vi "Hall_analysis_dataview.vi"(8 "Y-column names":string[](array[string])=["Kxy"], 10 "column extension":string[](array[string])=["NC", "C"], 11 "Graph array":cluster{"output":dbl[], "output":dbl[]}[](array[cluster])=[{"output"=[-18.0, -17.8, -17.5, -17.2, -16.9, -16.6, -16.3, -16.0, -15.7, -15.4, -15.1, -14.8, -14.5, -14.2, -13.9, -13.6, -13.3, -13.0, -12.7, -12.4, -12.1, -11.8, -11.5, -11.2, -10.9, -10.6, -10.3, -10.0, -9.7, -9.4, -9.2, -9.0, -8.8, -8.6, -8.4, -8.2, -8.0, -7.8, -7.6, -7.4, -7.2, -7.0, -6.8, -6.6, -6.4, -6.2, -6.0, -5.8, -5.6, -5.4, -5.2, -5.0, -4.8, -4.6, -4.4, -4.2, -4.1, -4.0, -3.9, -3.8, -3.7, -3.6, -3.5, -3.4, -3.3, -3.2, -3.1, -3.0, -2.9, -2.8, -2.7, -2.6, -2.5, -2.4, -2.3, -2.2, -2.1, -2.0, -1.9, -1.8, -1.7, -1.6, -1.5, -1.4, -1.3, -1.2, -1.1, -1.0, -0.9, -0.8, -0.7, -0.6, -0.5, -0.4, -0.3, -0.2, -0.1, 0.0, 0.1, 0.2, 0.3, 0.4, 0.5, 0.6, 0.6, 0.7, 0.7, 0.8, 0.8, 0.9, 0.9, 1.0, 1.0, 1.1, 1.1, 1.2, 1.2, 1.3, 1.3, 1.4, 1.4, 1.5, 1.5, 1.6, 1.6, 1.7, 1.7, 1.8, 1.8, 1.9, 1.9, 1.9, 2.0, 2.0, 2.0, 2.0, 2.1, 2.2, 2.3, 2.4, 2.5, 2.6, 2.7, 2.8, 2.9, 3.0, 3.1, 3.2, 3.3, 3.4, 3.5, 3.6, 3.7, 3.8, 3.9, 4.0, 4.1, 4.3, 4.5, 4.7, 4.9, 5.1, 5.3, 5.5, 5.7, 5.9, 6.1, 6.3, 6.5, 6.7, 6.9, 7.1, 7.3, 7.5, 7.7, 7.9, 8.1, 8.3, 8.5, 8.7, 8.9, 9.1, 9.3, 9.6, 9.9, 10.2, 10.5, 11.4, 11.7, 12.0, 12.3, 12.6, 12.9, 13.2, 13.5, 13.8, 14.1, 14.4, 14.7, 15.0, 15.3, 15.6, 15.9, 16.2, 16.5, 16.8, 17.1, 17.4, 17.7, 18.0], "output"=[0.054529, 0.058942, 0.066239, 0.077061, 0.087056, 0.10131, 0.11992, 0.1396, 0.16271, 0.18625, 0.2129, 0.23568, 0.26388, 0.29975, 0.34124, 0.37943, 0.3989, 0.44212, 0.48919, 0.5041, 0.54167, 0.58119, 0.59731, 0.60919, 0.66613, 0.66507, 0.71084, 0.72607, 0.72221, 0.74336, 0.77984, 0.77621, 0.77261, 0.80307, 0.76644, 0.80808, 0.81198, 0.81508, 0.79026, 0.84278, 0.81013, 0.81826, 0.84746, 0.83187, 0.83075, 0.83154, 0.81118, 0.84682, 0.85035, 0.83341, 0.83691, 0.79145, 0.83157, 0.83834, 0.80534, 0.81804, 0.82836, 0.82435, 0.78641, 0.75032, 0.7595, 0.77179, 0.77151, 0.778, 0.80644, 0.74695, 0.74781, 0.74014, 0.79086, 0.72817, 0.75592, 0.74425, 0.74898, 0.73582, 0.73516, 0.72155, 0.71542, 0.71347, 0.73071, 0.70282, 0.69885, 0.70647, 0.70025, 0.67747, 0.68127, 0.70861, 0.67626, 0.68964, 0.64825, 0.67411, 0.66336, 0.656, 0.65756, 0.67107, 0.70006, 0.698, 0.67342, 0.6801, 0.66464, 0.63203, 0.69444, 0.708, 0.69388, 0.7146, 0.66843, 0.74125, 0.64612, 0.73964, 0.62851, 0.7537, 0.66641, 0.72491, 0.69419, 0.73232, 0.67301, 0.72483, 0.68845, 0.76522, 0.69356, 0.72033, 0.67263, 0.73855, 0.67125, 0.77098, 0.74016, 0.74964, 0.69619, 0.77965, 0.75816, 0.76918, 0.73759, 0.77935, 0.78748, 0.81876, 0.77574, 0.73471, 0.81422, 0.78848, 0.82829, 0.80536, 0.78947, 0.79377, 0.78297, 0.81896, 0.83866, 0.84293, 0.84248, 0.85276, 0.85255, 0.83921, 0.86151, 0.84402, 0.87765, 0.84703, 0.84606, 0.86928, 0.83403, 0.86374, 0.84952, 0.87353, 0.85058, 0.86321, 0.84461, 0.88025, 0.872, 0.89059, 0.88649, 0.888, 0.88664, 0.86834, 0.88418, 0.87369, 0.82698, 0.83785, 0.8636, 0.86849, 0.84876, 0.84895, 0.86216, 0.85159, 0.77613, 0.81179, 0.80194, 0.77828, 0.80233, 0.73352, 0.7213, 0.63859, 0.62626, 0.60173, 0.57119, 0.51729, 0.48595, 0.42536, 0.4044, 0.36236, 0.32568, 0.28429, 0.25023, 0.22166, 0.19862, 0.1831, 0.14912, 0.12865, 0.11025, 0.094853, 0.081756, 0.070731, 0.062495, 0.055254]}, {"output"=[-18.0, -17.8, -17.5, -17.2, -16.9, -16.6, -16.3, -16.0, -15.7, -15.4, -15.1, -14.8, -14.5, -14.2, -13.9, -13.6, -13.3, -13.0, -12.7, -12.4, -12.1, -11.8, -11.5, -11.2, -10.9, -10.6, -10.3, -10.0, -9.7, -9.4, -9.2, -9.0, -8.8, -8.6, -8.4, -8.2, -8.0, -7.8, -7.6, -7.4, -7.2, -7.0, -6.8, -6.6, -6.4, -6.2, -6.0, -5.8, -5.6, -5.4, -5.2, -5.0, -4.8, -4.6, -4.4, -4.2, -4.1, -4.0, -3.9, -3.8, -3.7, -3.6, -3.5, -3.4, -3.3, -3.2, -3.1, -3.0, -2.9, -2.8, -2.7, -2.6, -2.5, -2.4, -2.3, -2.2, -2.1, -2.0, -1.9, -1.8, -1.7, -1.6, -1.5, -1.4, -1.3, -1.2, -1.1, -1.0, -0.9, -0.8, -0.7, -0.6, -0.5, -0.4, -0.3, -0.2, -0.1, 0.0, 0.0, 0.0, 0.0, 0.1, 0.1, 0.2, 0.2, 0.3, 0.3, 0.4, 0.4, 0.5, 0.5, 0.6, 0.6, 0.7, 0.7, 0.8, 0.8, 0.9, 0.9, 1.0, 1.0, 1.1, 1.1, 1.2, 1.2, 1.2, 1.3, 1.4, 1.4, 1.4, 1.5, 1.5, 1.5, 1.6, 1.6, 1.6, 1.7, 1.7, 1.7, 1.8, 1.8, 1.8, 1.9, 1.9, 1.9, 1.9, 2.0, 2.0, 2.0, 2.0, 2.0, 2.1, 2.2, 2.3, 2.4, 2.5, 2.6, 2.7, 2.8, 2.9, 3.0, 3.2, 3.3, 3.4, 3.5, 3.6, 3.7, 3.8, 3.9, 4.0, 4.1, 4.3, 4.5, 4.7, 4.9, 5.1, 5.3, 5.5, 5.7, 5.9, 6.1, 6.3, 6.5, 6.7, 6.9, 7.1, 7.3, 7.5, 7.7, 7.9, 8.1, 8.3, 8.5, 8.7, 8.9, 9.1, 9.3, 9.6, 9.9, 10.2, 10.5, 11.4, 11.7, 12.0, 12.3, 12.6, 12.9, 13.2, 13.5, 13.8, 14.1, 14.4, 14.7, 15.0, 15.3, 15.6, 15.9, 16.2, 16.5, 16.8, 17.1, 17.4, 17.7, 18.0], "output"=[0.04639503, 0.05124551, 0.05869006, 0.06889321, 0.07842688, 0.09168241, 0.1088334, 0.1275547, 0.1497657, 0.1728078, 0.1996734, 0.2230474, 0.252526, 0.2881616, 0.327736, 0.3626875, 0.3799339, 0.4162642, 0.4502874, 0.4540727, 0.4752561, 0.4913592, 0.4877077, 0.4808698, 0.5060909, 0.4841805, 0.4946125, 0.4869426, 0.4643427, 0.4633326, 0.475855, 0.4651067, 0.45418, 0.4655186, 0.439674, 0.4540213, 0.4526447, 0.452366, 0.4296351, 0.4631344, 0.4392119, 0.4478341, 0.4652855, 0.4548735, 0.4575837, 0.4587661, 0.4438654, 0.469387, 0.470055, 0.4578611, 0.4516406, 0.4175235, 0.436408, 0.4269168, 0.3872179, 0.3819697, 0.3767659, 0.3588841, 0.3260986, 0.2882154, 0.2814761, 0.2736725, 0.2563214, 0.2451817, 0.2437467, 0.1887873, 0.1645303, 0.1499105, 0.1638911, 0.1060275, 0.09419492, 0.06499817, 0.0570674, 0.02551558, 0.003708405, -0.02605604, -0.04799681, -0.06751369, -0.0846491, -0.1206419, -0.146525, -0.1597774, -0.1865335, -0.2201835, -0.2416687, -0.2474123, -0.2807871, -0.295045, -0.3360811, -0.3413561, -0.3589792, -0.3818877, -0.3994011, -0.4013593, -0.398709, -0.4129966, -0.4294426, -0.4040814, -0.4025437, -0.3969354, -0.4430137, -0.3701796, -0.4330835, -0.3728167, -0.4410564, -0.3769775, -0.400408, -0.3534563, -0.3830965, -0.3413242, -0.3789024, -0.3517245, -0.3759194, -0.3247219, -0.3729292, -0.3118913, -0.3624734, -0.2877669, -0.3256675, -0.2765885, -0.2927328, -0.2603341, -0.2851914, -0.2416307, -0.2405671, -0.2581909, -0.2354419, -0.1993335, -0.1469915, -0.2259791, -0.1720161, -0.3363505, -0.2092051, -0.1346528, -0.03116894, -0.1574943, -0.1216288, -0.2430438, -0.1582942, -0.08931337, -0.1297527, -0.1192861, -0.07149084, -0.1419238, -0.1457252, -0.09284115, -0.03720788, -0.102183, -0.1086995, -0.04796695, -0.104636, -0.00174423, 0.009173533, 0.05047776, 0.05254663, 0.07652015, 0.08893176, 0.1113383, 0.151861, 0.1836534, 0.1970177, 0.2455877, 0.2636115, 0.2712736, 0.3057058, 0.3097401, 0.3473493, 0.3425707, 0.3539546, 0.3803674, 0.3816536, 0.4126079, 0.4150657, 0.4464129, 0.44045, 0.4582221, 0.4505175, 0.4758656, 0.4795104, 0.4947396, 0.4848849, 0.4830822, 0.4786933, 0.4679154, 0.4795023, 0.4728305, 0.4473741, 0.4516747, 0.4679614, 0.4744294, 0.46412, 0.4744021, 0.487967, 0.4956767, 0.4472478, 0.4861927, 0.4899166, 0.4858326, 0.5285123, 0.5022734, 0.5113373, 0.5215333, 0.5057456, 0.4986291, 0.4954527, 0.4628171, 0.4464335, 0.3980344, 0.3780465, 0.3425009, 0.3082822, 0.2687738, 0.2353835, 0.2080937, 0.1842725, 0.1676573, 0.1364157, 0.1169751, 0.09968616, 0.0853419, 0.07318228, 0.06282505, 0.05469888, 0.0469797]}]) -> ()   [LabVIEW 2024]
uses:
  <vilib>/gmath/NI_Gmath.lvlib
panel:
  out "y-column name":string="Kxy_NCC"
  out "Hall data":cluster{"output":dbl[], "output":dbl[]}[](graph)=[{"output"=[-0.0, 0.3272743225097656, 0.6545467376708984, 0.9818191528320312, 1.309091567993164, 1.6363639831542969, 1.9636363983154297, 2.290909767150879, 2.6181821823120117, 2.945455551147461, 3.2727279663085938, 3.6000003814697266, 3.927273750305176, 4.254546165466309, 4.581818580627441, 4.909091949462891, 5.236364364624023, 5.563636779785156, 5.890909194946289, 6.218182563781738, 6.545454978942871, 6.872727394104004, 7.200000762939453, 7.527273178100586, 7.854545593261719, 8.181818962097168, 8.5090913772583, 8.836363792419434, 9.163637161254883, 9.490909576416016, 9.818181991577148, 10.145454406738281, 10.47272777557373, 10.800000190734863, 11.127273559570312, 11.454545974731445, 11.781818389892578, 12.109090805053711, 12.436363220214844, 12.763636589050293, 13.090909957885742, 13.418182373046875, 13.745454788208008, 14.07272720336914, 14.399999618530273, 14.727272987365723, 15.054545402526855, 15.381818771362305, 15.709091186523438, 16.03636360168457, 16.363636016845703, 16.690908432006836, 17.0181827545166, 17.345455169677734, 17.672727584838867, 18.0], "output"=[0.0, 0.00299248279571529, -0.0018767957687377823, 0.003511941719055167, 0.0053665068054198906, 0.010236265392303434, 0.008009093399047817, 0.04537398966789241, 0.022717283315658587, 0.03639796306610105, 0.031195704059600815, 0.03611515687942507, 0.027817319812774688, 0.021205686359405507, 0.012001070156097415, 0.020733940610885626, 0.007127333927154533, 0.01517751313209531, 0.029562425460815445, 0.027957046141624475, 0.025458204402923568, 0.02258906681060785, 0.020102571363449062, 0.016001556339263923, 0.026572024908065817, 0.020201597528457627, 0.037629742684364365, 0.01343787633895871, 0.014737974634170536, 0.024966436818440796, 0.03602008089701325, 0.013672806886037503, 0.018961714207331226, 0.013976701386769541, 0.020330128383636348, 0.018619129714965765, 0.018701590213775487, 0.025046611016591225, 0.022198663406372054, 0.010495055723190427, 0.009185015996297174, 0.009443247070312494, 0.004545132083892844, 0.005831363080342794, 0.0042268017514546785, 0.002558227068583274, 0.0005598068555196234, 0.003261120878855439, 0.004366964670816931, 0.0013005196634929411, 0.0013206059392292177, 0.001730701716105211, 0.0011047034600575323, 0.00046085776265467754, 0.0006030408445993653, 0.00036249999999999824]}, {"output"=[-0.0, 0.3272743225097656, 0.6545467376708984, 0.9818191528320312, 1.309091567993164, 1.6363639831542969, 1.9636363983154297, 2.290909767150879, 2.6181821823120117, 2.945455551147461, 3.2727279663085938, 3.6000003814697266, 3.927273750305176, 4.254546165466309, 4.581818580627441, 4.909091949462891, 5.236364364624023, 5.563636779785156, 5.890909194946289, 6.218182563781738, 6.545454978942871, 6.872727394104004, 7.200000762939453, 7.527273178100586, 7.854545593261719, 8.181818962097168, 8.5090913772583, 8.836363792419434, 9.163637161254883, 9.490909576416016, 9.818181991577148, 10.145454406738281, 10.47272777557373, 10.800000190734863, 11.127273559570312, 11.454545974731445, 11.781818389892578, 12.109090805053711, 12.436363220214844, 12.763636589050293, 13.090909957885742, 13.418182373046875, 13.745454788208008, 14.07272720336914, 14.399999618530273, 14.727272987365723, 15.054545402526855, 15.381818771362305, 15.709091186523438, 16.03636360168457, 16.363636016845703, 16.690908432006836, 17.0181827545166, 17.345455169677734, 17.672727584838867, 18.0], "output"=[0.0, 0.0018725577600479104, -0.0024482699415207254, 0.0018922374864578095, 0.0025667974205016986, -0.0168217872724533, -0.024209317914752962, 0.022859984019057276, 0.011349383976507185, 0.01609591005096435, 0.01496877274971009, 0.018033754336547858, 0.013058585019016272, 0.011085874159431464, 0.0022907896628856783, 0.007575240142726897, 9.869320383074087e-05, 0.004593664635086064, 0.018130483435058575, 0.012580532687187201, 0.010315582862472528, 0.009491347095203384, 0.010445227202796947, 0.00603945345125198, 0.010258666759109497, 0.007215023374080642, 0.01727315357503889, 0.0032452536701679524, 0.006738375054264056, 0.011839508860651687, 0.021813215582338813, 0.00819147609920512, 0.010953557992998797, 0.007974255379909978, 0.015729827381049277, 0.015995607844606963, 0.006333438585472084, 0.011429940308507275, 0.013502250313059488, 0.005405149334716863, 0.005189663690376267, 0.0051790019136429, 0.0016113218469619717, 0.0032211251384736683, 0.00218476138941448, 0.0013544852338791824, 0.00027394241498311656, 0.002652594708252007, 0.0036020352183022963, 0.0011468679021836292, 0.0011747290191267898, 0.0014462527038765494, 0.0009137086473528164, 0.0003810429619217487, 0.0005169348717689037, 0.0002923350000000012]}]
  in  "Data analyis method":T1(ring)
  in  "smooth":bool=TRUE
  in  "smooth factor":i32=1
  in  "iteration Number":i32=1
  in  "interpolation size":u16=111 min=1 step=1
  in  "max H":sgl=18.0 min=0 format="%.2f"
  in  "export":T2(ring)=enum."write to clipboard"
  out "raw data":cluster{"all rows":dbl[], "all rows":dbl[]}[](graph)=[{"all rows"=[-18.0, -17.8, -17.5, -17.2, -16.9, -16.6, -16.3, -16.0, -15.7, -15.4, -15.1, -14.8, -14.5, -14.2, -13.9, -13.6, -13.3, -13.0, -12.7, -12.4, -12.1, -11.8, -11.5, -11.2, -10.9, -10.6, -10.3, -10.0, -9.7, -9.4, -9.2, -9.0, -8.8, -8.6, -8.4, -8.2, -8.0, -7.8, -7.6, -7.4, -7.2, -7.0, -6.8, -6.6, -6.4, -6.2, -6.0, -5.8, -5.6, -5.4, -5.2, -5.0, -4.8, -4.6, -4.4, -4.2, -4.1, -4.0, -3.9, -3.8, -3.7, -3.6, -3.5, -3.4, -3.3, -3.2, -3.1, -3.0, -2.9, -2.8, -2.7, -2.6, -2.5, -2.4, -2.3, -2.2, -2.1, -2.0, -1.9, -1.8, -1.7, -1.6, -1.5, -1.4, -1.3, -1.2, -1.1, -1.0, -0.9, -0.8, -0.7, -0.6, -0.5, -0.4, -0.3, -0.2, -0.1, 0.0, 0.1, 0.2, 0.3, 0.4, 0.5, 0.6, 0.6, 0.7, 0.7, 0.8, 0.8, 0.9, 0.9, 1.0, 1.0, 1.1, 1.1, 1.2, 1.2, 1.3, 1.3, 1.4, 1.4, 1.5, 1.5, 1.6, 1.6, 1.7, 1.7, 1.8, 1.8, 1.9, 1.9, 1.9, 2.0, 2.0, 2.0, 2.0, 2.1, 2.2, 2.3, 2.4, 2.5, 2.6, 2.7, 2.8, 2.9, 3.0, 3.1, 3.2, 3.3, 3.4, 3.5, 3.6, 3.7, 3.8, 3.9, 4.0, 4.1, 4.3, 4.5, 4.7, 4.9, 5.1, 5.3, 5.5, 5.7, 5.9, 6.1, 6.3, 6.5, 6.7, 6.9, 7.1, 7.3, 7.5, 7.7, 7.9, 8.1, 8.3, 8.5, 8.7, 8.9, 9.1, 9.3, 9.6, 9.9, 10.2, 10.5, 11.4, 11.7, 12.0, 12.3, 12.6, 12.9, 13.2, 13.5, 13.8, 14.1, 14.4, 14.7, 15.0, 15.3, 15.6, 15.9, 16.2, 16.5, 16.8, 17.1, 17.4, 17.7, 18.0], "all rows"=[0.054529, 0.058942, 0.066239, 0.077061, 0.087056, 0.10131, 0.11992, 0.1396, 0.16271, 0.18625, 0.2129, 0.23568, 0.26388, 0.29975, 0.34124, 0.37943, 0.3989, 0.44212, 0.48919, 0.5041, 0.54167, 0.58119, 0.59731, 0.60919, 0.66613, 0.66507, 0.71084, 0.72607, 0.72221, 0.74336, 0.77984, 0.77621, 0.77261, 0.80307, 0.76644, 0.80808, 0.81198, 0.81508, 0.79026, 0.84278, 0.81013, 0.81826, 0.84746, 0.83187, 0.83075, 0.83154, 0.81118, 0.84682, 0.85035, 0.83341, 0.83691, 0.79145, 0.83157, 0.83834, 0.80534, 0.81804, 0.82836, 0.82435, 0.78641, 0.75032, 0.7595, 0.77179, 0.77151, 0.778, 0.80644, 0.74695, 0.74781, 0.74014, 0.79086, 0.72817, 0.75592, 0.74425, 0.74898, 0.73582, 0.73516, 0.72155, 0.71542, 0.71347, 0.73071, 0.70282, 0.69885, 0.70647, 0.70025, 0.67747, 0.68127, 0.70861, 0.67626, 0.68964, 0.64825, 0.67411, 0.66336, 0.656, 0.65756, 0.67107, 0.70006, 0.698, 0.67342, 0.6801, 0.66464, 0.63203, 0.69444, 0.708, 0.69388, 0.7146, 0.66843, 0.74125, 0.64612, 0.73964, 0.62851, 0.7537, 0.66641, 0.72491, 0.69419, 0.73232, 0.67301, 0.72483, 0.68845, 0.76522, 0.69356, 0.72033, 0.67263, 0.73855, 0.67125, 0.77098, 0.74016, 0.74964, 0.69619, 0.77965, 0.75816, 0.76918, 0.73759, 0.77935, 0.78748, 0.81876, 0.77574, 0.73471, 0.81422, 0.78848, 0.82829, 0.80536, 0.78947, 0.79377, 0.78297, 0.81896, 0.83866, 0.84293, 0.84248, 0.85276, 0.85255, 0.83921, 0.86151, 0.84402, 0.87765, 0.84703, 0.84606, 0.86928, 0.83403, 0.86374, 0.84952, 0.87353, 0.85058, 0.86321, 0.84461, 0.88025, 0.872, 0.89059, 0.88649, 0.888, 0.88664, 0.86834, 0.88418, 0.87369, 0.82698, 0.83785, 0.8636, 0.86849, 0.84876, 0.84895, 0.86216, 0.85159, 0.77613, 0.81179, 0.80194, 0.77828, 0.80233, 0.73352, 0.7213, 0.63859, 0.62626, 0.60173, 0.57119, 0.51729, 0.48595, 0.42536, 0.4044, 0.36236, 0.32568, 0.28429, 0.25023, 0.22166, 0.19862, 0.1831, 0.14912, 0.12865, 0.11025, 0.094853, 0.081756, 0.070731, 0.062495, 0.055254]}, {"all rows"=[-18.0, -17.8, -17.5, -17.2, -16.9, -16.6, -16.3, -16.0, -15.7, -15.4, -15.1, -14.8, -14.5, -14.2, -13.9, -13.6, -13.3, -13.0, -12.7, -12.4, -12.1, -11.8, -11.5, -11.2, -10.9, -10.6, -10.3, -10.0, -9.7, -9.4, -9.2, -9.0, -8.8, -8.6, -8.4, -8.2, -8.0, -7.8, -7.6, -7.4, -7.2, -7.0, -6.8, -6.6, -6.4, -6.2, -6.0, -5.8, -5.6, -5.4, -5.2, -5.0, -4.8, -4.6, -4.4, -4.2, -4.1, -4.0, -3.9, -3.8, -3.7, -3.6, -3.5, -3.4, -3.3, -3.2, -3.1, -3.0, -2.9, -2.8, -2.7, -2.6, -2.5, -2.4, -2.3, -2.2, -2.1, -2.0, -1.9, -1.8, -1.7, -1.6, -1.5, -1.4, -1.3, -1.2, -1.1, -1.0, -0.9, -0.8, -0.7, -0.6, -0.5, -0.4, -0.3, -0.2, -0.1, 0.0, 0.0, 0.0, 0.0, 0.1, 0.1, 0.2, 0.2, 0.3, 0.3, 0.4, 0.4, 0.5, 0.5, 0.6, 0.6, 0.7, 0.7, 0.8, 0.8, 0.9, 0.9, 1.0, 1.0, 1.1, 1.1, 1.2, 1.2, 1.2, 1.3, 1.4, 1.4, 1.4, 1.5, 1.5, 1.5, 1.6, 1.6, 1.6, 1.7, 1.7, 1.7, 1.8, 1.8, 1.8, 1.9, 1.9, 1.9, 1.9, 2.0, 2.0, 2.0, 2.0, 2.0, 2.1, 2.2, 2.3, 2.4, 2.5, 2.6, 2.7, 2.8, 2.9, 3.0, 3.2, 3.3, 3.4, 3.5, 3.6, 3.7, 3.8, 3.9, 4.0, 4.1, 4.3, 4.5, 4.7, 4.9, 5.1, 5.3, 5.5, 5.7, 5.9, 6.1, 6.3, 6.5, 6.7, 6.9, 7.1, 7.3, 7.5, 7.7, 7.9, 8.1, 8.3, 8.5, 8.7, 8.9, 9.1, 9.3, 9.6, 9.9, 10.2, 10.5, 11.4, 11.7, 12.0, 12.3, 12.6, 12.9, 13.2, 13.5, 13.8, 14.1, 14.4, 14.7, 15.0, 15.3, 15.6, 15.9, 16.2, 16.5, 16.8, 17.1, 17.4, 17.7, 18.0], "all rows"=[0.04639503, 0.05124551, 0.05869006, 0.06889321, 0.07842688, 0.09168241, 0.1088334, 0.1275547, 0.1497657, 0.1728078, 0.1996734, 0.2230474, 0.252526, 0.2881616, 0.327736, 0.3626875, 0.3799339, 0.4162642, 0.4502874, 0.4540727, 0.4752561, 0.4913592, 0.4877077, 0.4808698, 0.5060909, 0.4841805, 0.4946125, 0.4869426, 0.4643427, 0.4633326, 0.475855, 0.4651067, 0.45418, 0.4655186, 0.439674, 0.4540213, 0.4526447, 0.452366, 0.4296351, 0.4631344, 0.4392119, 0.4478341, 0.4652855, 0.4548735, 0.4575837, 0.4587661, 0.4438654, 0.469387, 0.470055, 0.4578611, 0.4516406, 0.4175235, 0.436408, 0.4269168, 0.3872179, 0.3819697, 0.3767659, 0.3588841, 0.3260986, 0.2882154, 0.2814761, 0.2736725, 0.2563214, 0.2451817, 0.2437467, 0.1887873, 0.1645303, 0.1499105, 0.1638911, 0.1060275, 0.09419492, 0.06499817, 0.0570674, 0.02551558, 0.003708405, -0.02605604, -0.04799681, -0.06751369, -0.0846491, -0.1206419, -0.146525, -0.1597774, -0.1865335, -0.2201835, -0.2416687, -0.2474123, -0.2807871, -0.295045, -0.3360811, -0.3413561, -0.3589792, -0.3818877, -0.3994011, -0.4013593, -0.398709, -0.4129966, -0.4294426, -0.4040814, -0.4025437, -0.3969354, -0.4430137, -0.3701796, -0.4330835, -0.3728167, -0.4410564, -0.3769775, -0.400408, -0.3534563, -0.3830965, -0.3413242, -0.3789024, -0.3517245, -0.3759194, -0.3247219, -0.3729292, -0.3118913, -0.3624734, -0.2877669, -0.3256675, -0.2765885, -0.2927328, -0.2603341, -0.2851914, -0.2416307, -0.2405671, -0.2581909, -0.2354419, -0.1993335, -0.1469915, -0.2259791, -0.1720161, -0.3363505, -0.2092051, -0.1346528, -0.03116894, -0.1574943, -0.1216288, -0.2430438, -0.1582942, -0.08931337, -0.1297527, -0.1192861, -0.07149084, -0.1419238, -0.1457252, -0.09284115, -0.03720788, -0.102183, -0.1086995, -0.04796695, -0.104636, -0.00174423, 0.009173533, 0.05047776, 0.05254663, 0.07652015, 0.08893176, 0.1113383, 0.151861, 0.1836534, 0.1970177, 0.2455877, 0.2636115, 0.2712736, 0.3057058, 0.3097401, 0.3473493, 0.3425707, 0.3539546, 0.3803674, 0.3816536, 0.4126079, 0.4150657, 0.4464129, 0.44045, 0.4582221, 0.4505175, 0.4758656, 0.4795104, 0.4947396, 0.4848849, 0.4830822, 0.4786933, 0.4679154, 0.4795023, 0.4728305, 0.4473741, 0.4516747, 0.4679614, 0.4744294, 0.46412, 0.4744021, 0.487967, 0.4956767, 0.4472478, 0.4861927, 0.4899166, 0.4858326, 0.5285123, 0.5022734, 0.5113373, 0.5215333, 0.5057456, 0.4986291, 0.4954527, 0.4628171, 0.4464335, 0.3980344, 0.3780465, 0.3425009, 0.3082822, 0.2687738, 0.2353835, 0.2080937, 0.1842725, 0.1676573, 0.1364157, 0.1169751, 0.09968616, 0.0853419, 0.07318228, 0.06282505, 0.05469888, 0.0469797]}]
  in  "stop":bool
  in  "export Hall data":bool
  # "Fitting is done for the range given by 'Bbkg init' and 'Bbkg final'.\nBackground curve is extended to the range give by 'B init' and 'B final'.\nFFT is done in the range given by 'B init' and 'B final'."
  # "Also removes NaN"
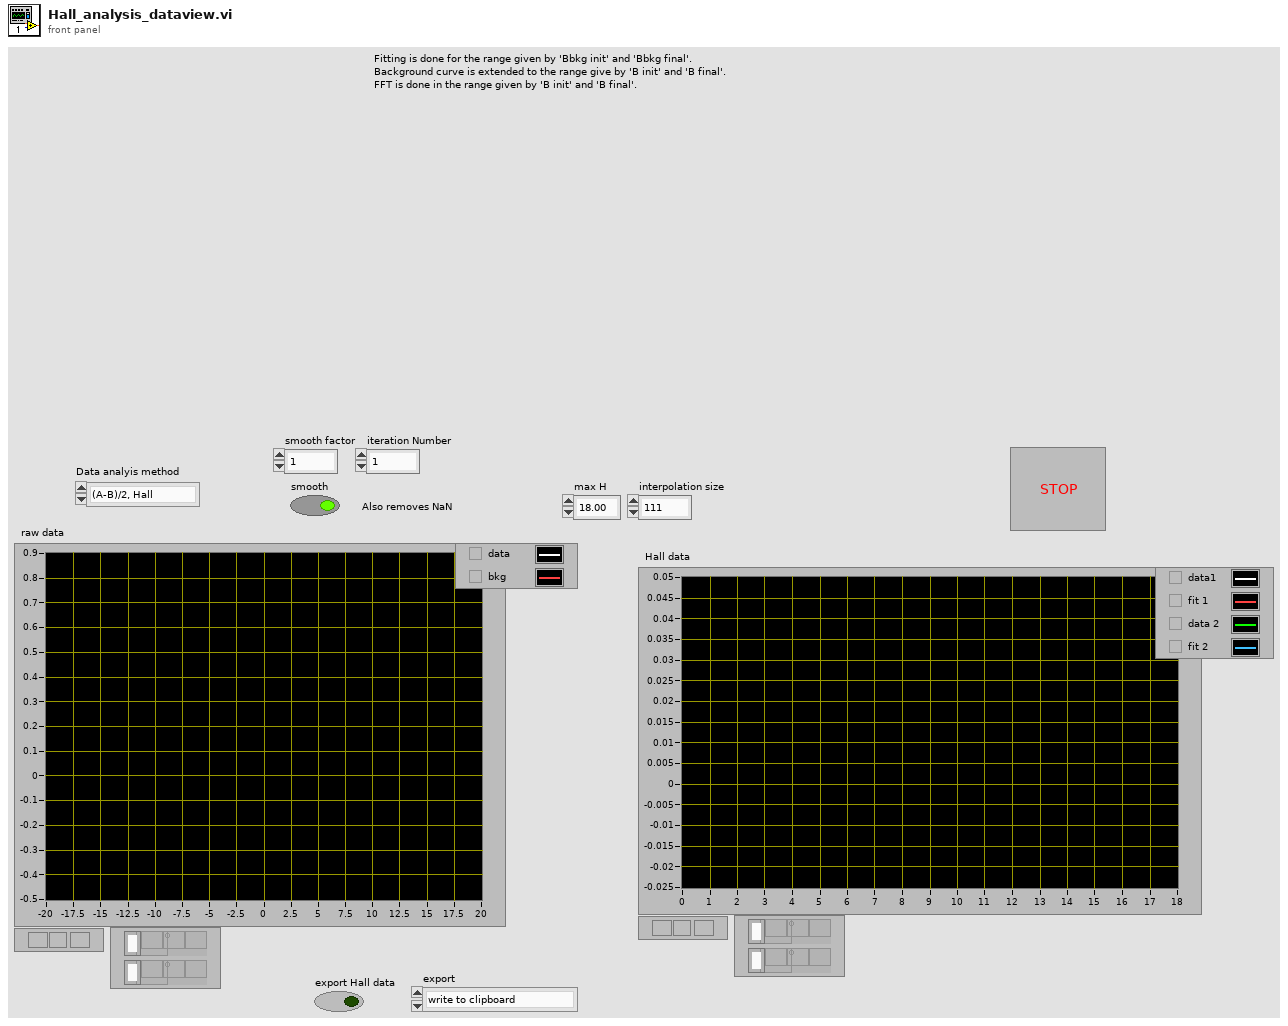
[diagram p1: front panel]
types:
  T1 = enum16{"(A-B)/2, Hall", "(A+B)/2, MR", "diagram defined"}
  T2 = enum16{"Save as Ascill file", "write to clipboard", "write to Igor ITX file"}
  T3 = enum16{"Save as Ascill file", "write to clipboard", "do not export"}
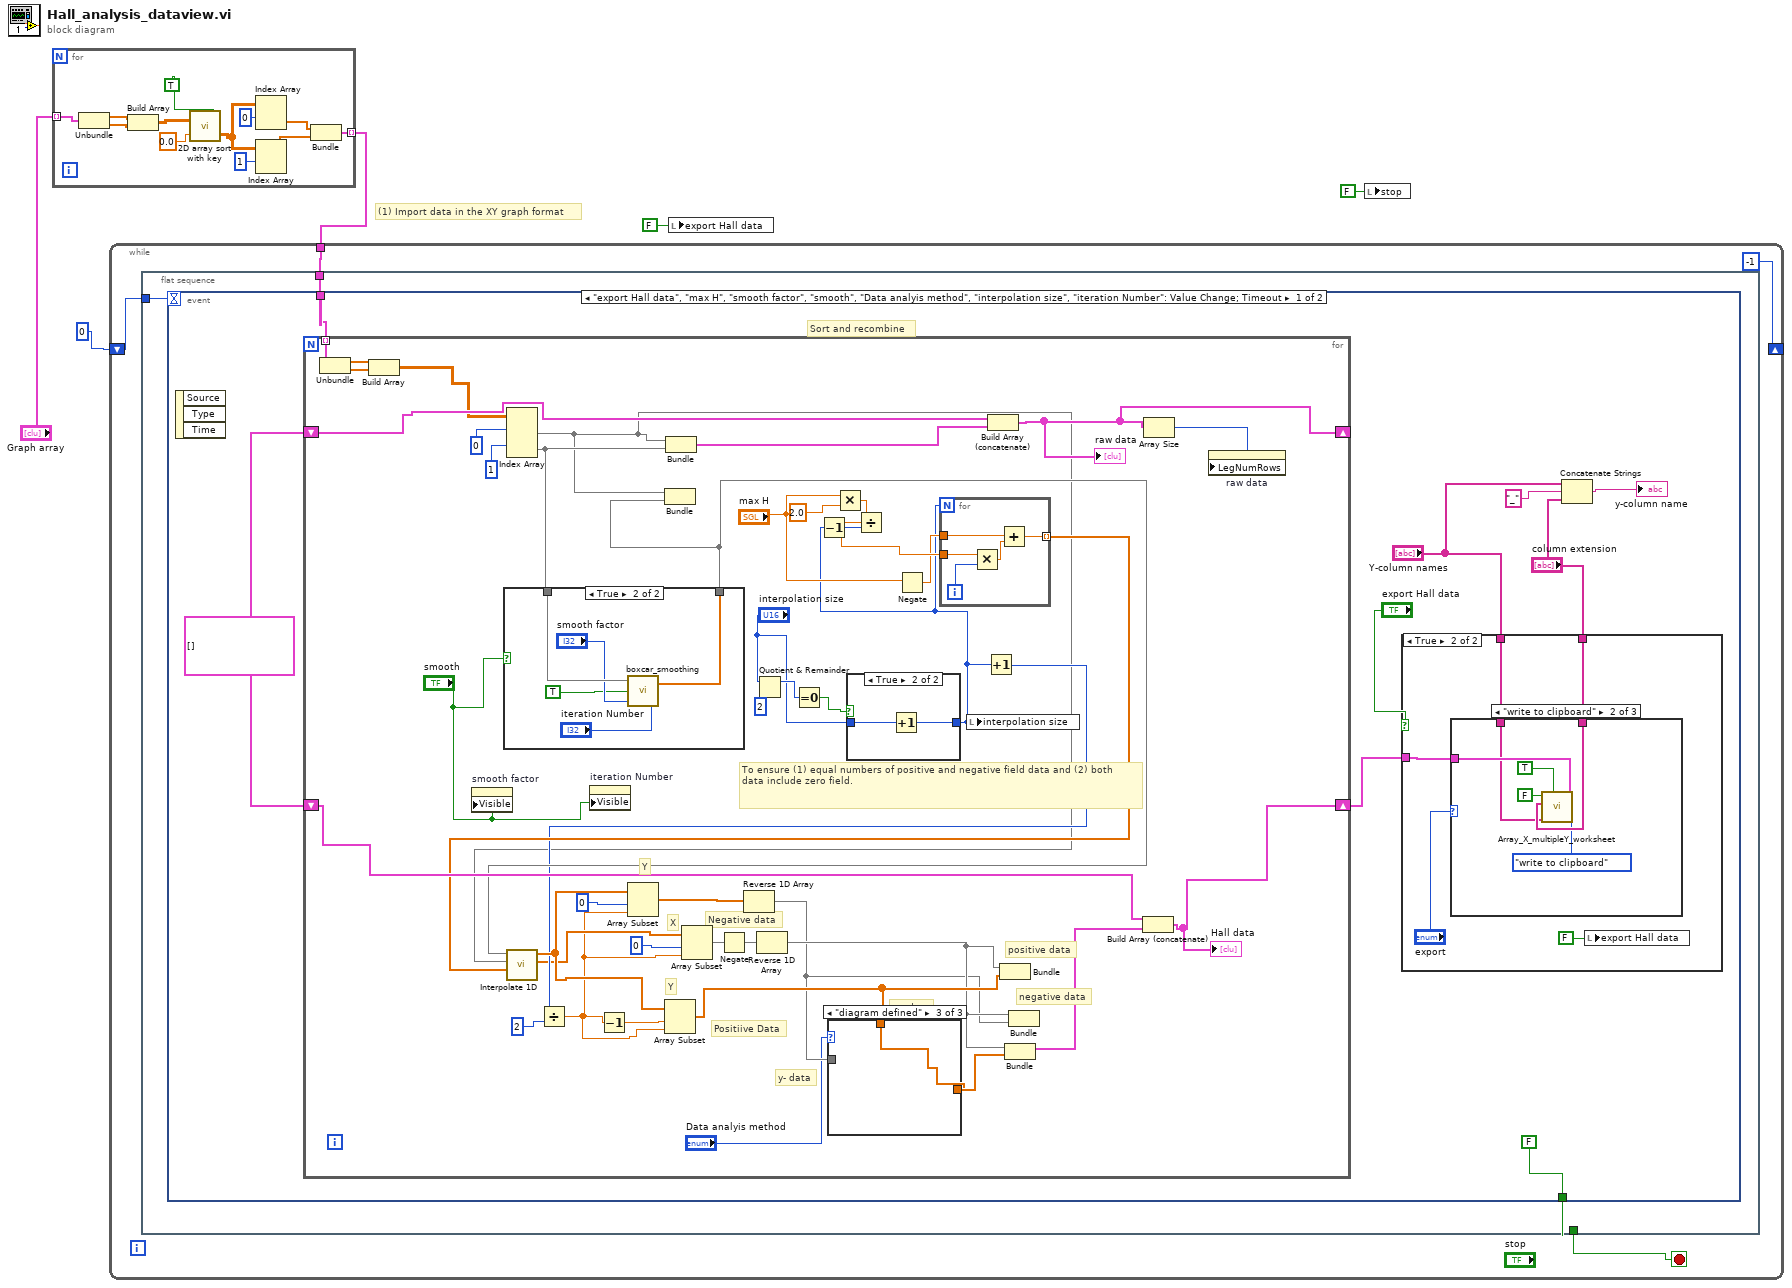
[diagram p0: block diagram]
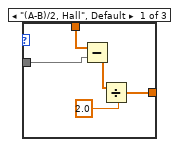
[diagram p3: hidden frame]
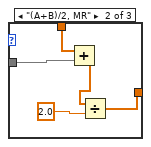
[diagram p4: hidden frame]
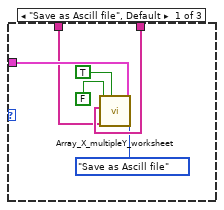
[diagram p7: hidden frame]
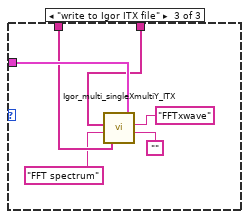
[diagram p8: hidden frame]
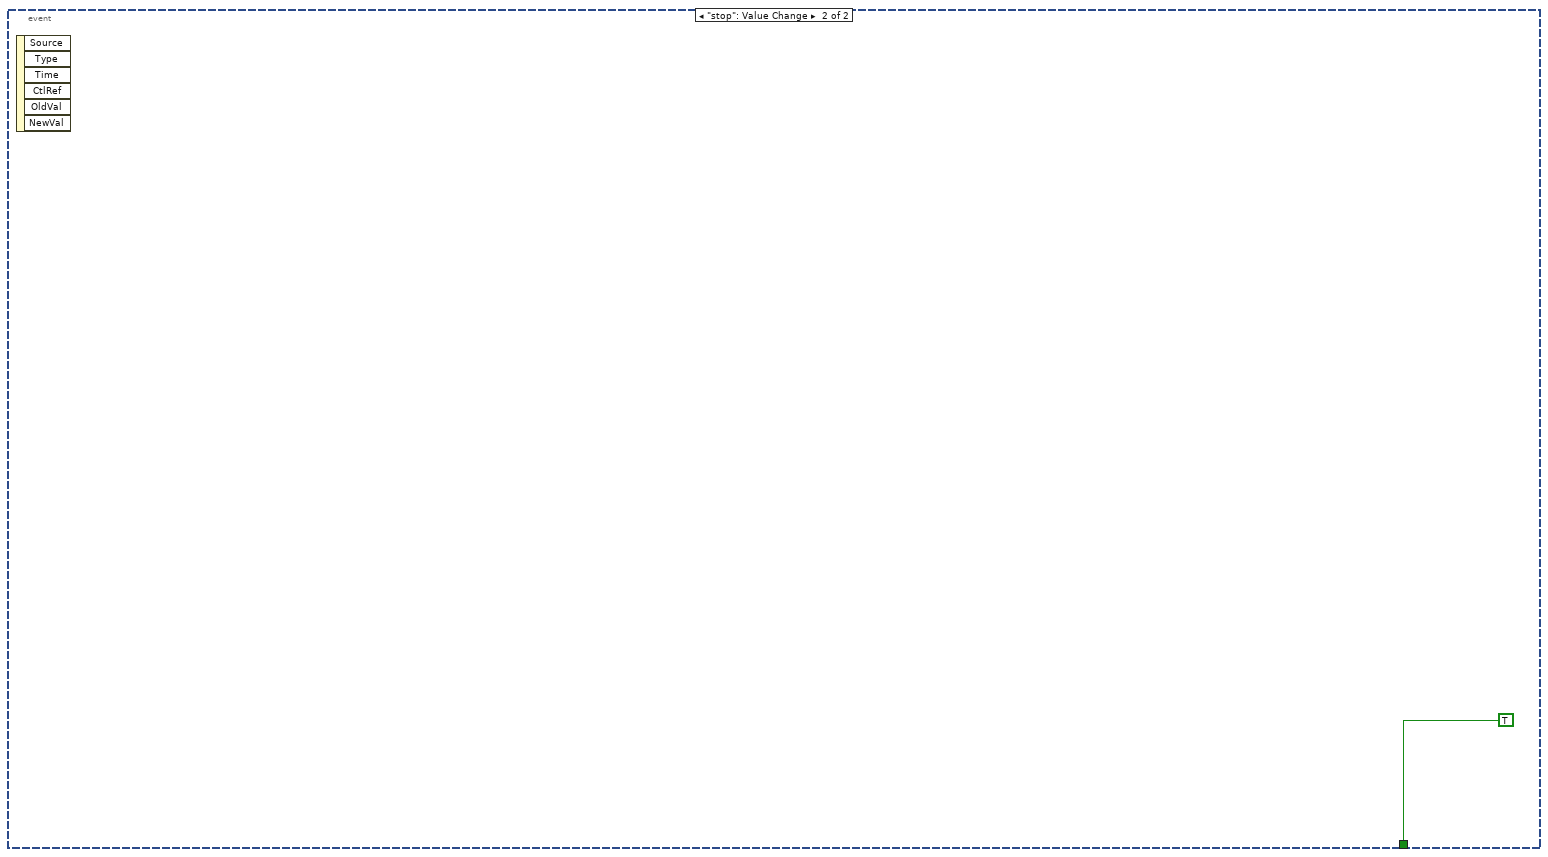
[diagram p9: hidden frame]
diagram:
  # "(1) Import data in the XY graph format"
  n1 = for {
    tunnel: "Graph array" -> [w17] mode=indexing
    tunnel: [w6] -> w4 mode=indexing
    n2 = Unbundle(w17) -> ("output"=w15:dbl[], "output"=w14:dbl[])
    n3 = Build Array(w15, w14) -> (w13:dbl[][])
    n4 = call "2D array sort with key.vi"("ascending"=TRUE, "key row"=0.0, "input"=w13) -> ("output"=w11:dbl[][])
    n5 = Index Array(array=w11, index (row)=0) -> (element=w8:dbl[])  [unwired: 1 in]
    n6 = Index Array(array=w11, index (row)=1) -> (element=w7:dbl[])  [unwired: 1 in]
    n7 = Bundle("output"=w8, "output"=w7) -> (w6:cluster{"output":dbl[], "output":dbl[]})  [unwired: 1 in]
  }
  n8 = while {
    tunnel: w4 -> [w21]
    shift-right: [-1] -> _
    shift-left: 0 -> [w19]
    stop <- w20 stop-if-true
    n9 = flat-sequence {
      tunnel: w21 -> [w24]
      tunnel: [w23] -> w20
      tunnel: w19 -> [w22]
      frame #0 {
        n10 = event shown="[0] \"export Hall data\", \"max H\", \"smooth factor\", \"smooth\", \"Data analyis method\", \"interpolation size\", \"iteration Number\": Value Change;  Timeout" {
          selector: _ -> [_ _]
          dyn-events: _ -> [_ _]
          timeout: w22 -> [_ _]
          tunnel: w24 -> [w32 _]
          tunnel: [FALSE ("stop (press twice)") TRUE ("stop (press twice)")] -> w23
          event "export Hall data", "max H", "smooth factor", "smooth", "Data analyis method", "interpolation size", "iteration Number": Value Change; Timeout {
            w25 = cluster{"all rows":sgl[], "all rows":sgl[]}[] []
            n11 = event-data() -> ()  [unwired: 1 in, 3 out]
            n12 = for {
              shift-right: [w73] -> w30
              shift-left: w25 -> [w74]
              tunnel: w32 -> [w78] mode=indexing
              shift-right: [w72] -> _
              shift-left: w25 -> [w75]
              # "negative data"
              # "positive data"
              # "y- data"
              # "Y"
              # "X"
              # "Y"
              # "Negative data"
              # "Positiive Data"
              # "To ensure (1) equal numbers of positive and negative field data and (2) both\ndata include zero field."
              # "y+ data"
              # "Sort and recombine"
              n13 = Unbundle(w78) -> ("output"=w77:dbl[], "output"=w76:dbl[])
              n14 = Build Array(w77, w76) -> (w34:dbl[][])
              n15 = property on="smooth factor" class="DigNum (strict)"("Visible"="smooth") -> ()  [unwired: 2 in, 2 out]
              n16 = Index Array(array=w34, index (row) #1=0 ("disabled index (col)"), index (row) #2=1 ("index (col)")) -> (element #1=w38:dbl[], element #2=w70:dbl[])  [unwired: 2 in]
              n17 = case shown="True" "smooth" {
                tunnel: w70 -> [w98 w103]
                tunnel: [w98 w102] -> w61
                frame False {
                }
                frame True {
                  n18 = call "boxcar_smoothing.vi"("iteration Number"="iteration Number", "smooth factor"="smooth factor", "remonve NaN"=TRUE, "raw data"=w103) -> ("smoothed"=w102:dbl[])
                }
              }
              n19 = property on="iteration Number" class="DigNum (strict)"("Visible"="smooth") -> ()  [unwired: 2 in, 2 out]
              n20 = Bundle(w38, "smoothed"=w61) -> ()  [unwired: 2 out]
              n21 = Bundle(w38, w70) -> (w37:cluster{dbl[], dbl[]})  [unwired: 1 out]
              n22 = Quotient & Remainder(x="interpolation size", y=u16 2) -> (x-y*floor(x/y)=w54:u16)  [unwired: 1 out]
              n23 = Equal To 0?(x=w54) -> (x = 0?=w55:bool)
              n24 = Multiply(x="max H", y=sgl 2.0) -> (x*y=w66:sgl)
              n25 = case shown="True" w55 {
                tunnel: "interpolation size" -> [w79 w81]
                tunnel: [w79 w80] -> w53
                frame False {
                }
                frame True {
                  n26 = Increment(x=w81) -> (x+1=w80:u16)
                }
              }
              n27 = Decrement(x=w53) -> (x-1=w40:u16)
              n28 = Divide(x=w66, y=w40) -> (x/y=w65:sgl)
              n29 = Negate(x="max H") -> (-x=w63:sgl)
              n30 = for {
                N: w53 -> [_]
                tunnel: w65 -> [w85]
                tunnel: w63 -> [w83]
                tunnel: [w82] -> w62 mode=indexing
                i -> [w86]
                n31 = Multiply(x=w85, y=w86) -> (x*y=w84:sgl)
                n32 = Add(x=w83, y=w84) -> (x+y=w82:sgl)
              }
              n33 = call <vilib>:"Interpolate 1D.vi"("xi"=w62, "X"=w38, "Y"=w61) -> ("xi used"=w51:dbl[], "yi"=w57:dbl[])  [unwired: 6 in, 1 out]
              n34 = local write "interpolation size"(w53) -> ()
              n35 = Increment(x=w53) -> (x+1=w52:u16)
              n36 = Divide(x=w52, y=u16 2) -> (x/y=w49:dbl)
              n37 = Decrement(x=w49) -> (x-1=w50:dbl)
              n38 = Array Subset(array=w57, index=0, length=w49) -> (w47:dbl[])
              n39 = Array Subset(array=w57, index=w50, length=w49) -> (w45:dbl[])
              n40 = Array Subset(array=w51, index=0, length=w49) -> (w48:dbl[])
              n41 = Negate(x=w48) -> (-x=w46:dbl[])
              n42 = Reverse 1D Array(array=w47) -> (reversed array=w43:dbl[])
              n43 = Reverse 1D Array(array=w46) -> (reversed array=w44:dbl[])
              n44 = case shown="\"diagram defined\"" "Data analyis method" {
                tunnel: w45 -> [w91 w96 w97]
                tunnel: w43 -> [w88 w93 _]
                tunnel: [w87 w92 w97] -> w42
                frame "(A-B)/2, Hall", Default {
                  n45 = Subtract(x=w91, y=w88) -> (x-y=w89:dbl[])
                  n46 = Divide(x=w89, y=2.0) -> (x/y=w87:dbl[])
                }
                frame "(A+B)/2, MR" {
                  n47 = Add(x=w96, y=w93) -> (x+y=w94:dbl[])
                  n48 = Divide(x=w94, y=2.0) -> (x/y=w92:dbl[])
                }
                frame "diagram defined" {
                }
              }
              n49 = Build Array (concatenate)(w75, w37) -> (w72:cluster{"all rows":dbl[], "all rows":dbl[]}[])
              "raw data" <- w72
              n50 = Bundle(w44, w45) -> ()  [unwired: 2 out]
              n51 = Bundle(w44, w42) -> (w35:cluster{dbl[], dbl[]})  [unwired: 1 out]
              n52 = Bundle(w44, w43) -> ()  [unwired: 2 out]
              n53 = Build Array (concatenate)(w74, w35) -> (w73:cluster{"all rows":dbl[], "all rows":dbl[]}[])
              "Hall data" <- w73
              n54 = Array Size(array=w72) -> (size(s)=w36:i32)
              n55 = property on="raw data" class="XYGraph (strict)"("LegNumRows"=w36) -> ()  [unwired: 2 in, 2 out]
            }
            n56 = case shown="True" "export Hall data" {
              tunnel: w30 -> [_ w107]
              tunnel: "Y-column names" -> [_ w105]
              tunnel: "column extension" -> [_ w104]
              frame False {
              }
              frame True {
                n57 = case shown="\"write to clipboard\"" "export" {
                  tunnel: w107 -> [w114 w120 w126]
                  tunnel: w104 -> [w112 w118 w125]
                  tunnel: w105 -> [w111 w117 w124]
                  frame "Save as Ascill file", Default {
                    n58 = call "Array_X_multipleY_worksheet.vi"("export"=T3."Save as Ascill file", "graph file"=w114, "same x-data"=TRUE, "Y-column names"=w111, "column extension"=w112, "Sort?"=FALSE) -> ()  [unwired: 2 in, 2 out]
                  }
                  frame "write to clipboard" {
                    n59 = call "Array_X_multipleY_worksheet.vi"("export"=T3."write to clipboard", "graph file"=w120, "same x-data"=TRUE, "Y-column names"=w117, "column extension"=w118, "Sort?"=FALSE) -> ()  [unwired: 2 in, 2 out]
                  }
                  frame "write to Igor ITX file" {
                    n60 = call "Igor_multi_singleXmultiY_ITX.vi"("message"="", "x-column name"="FFTxwave", "graph file"=w126, "Y-column names"=w124, "window name"="FFT spectrum", "column extension"=w125) -> ()  [unwired: 1 in, 1 out]
                  }
                }
                n61 = local write "export Hall data"(FALSE ("export spectrum")) -> ()
              }
            }
            n62 = Concatenate Strings("Y-column names", "_" ("column_extension"), "column extension") -> (→"y-column name":string)
          }
          event "stop": Value Change {
            n63 = event-data() -> ()  [unwired: 1 in, 6 out]
          }
        }
      }
    }
  }
  n64 = local write "export Hall data"(FALSE ("export spectrum")) -> ()
  n65 = local write "stop"(FALSE ("stop")) -> ()
